vi "Write Return File Path Msg.vi"(10 "Return File Path Msg":refnum<class "Return File Path Msg.lvclass">, 11 "File Dialog in":refnum<class "File Dialog.lvclass">) -> (3 "File Dialog out":refnum<class "File Dialog.lvclass">)   [LabVIEW 2018, in "File Dialog Actor.lvlib" / "File Dialog.lvclass"]
uses:
  File Dialog.lvclass
  File Dialog Messages/Return File Path Msg/Return File Path Msg.lvclass
  File Dialog.lvclass/File Dialog.ctl
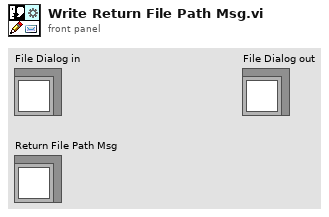
[diagram p1: front panel]
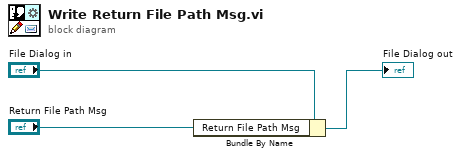
[diagram p0: block diagram]
diagram:
  n1 = Bundle By Name(cluster="File Dialog in", "Return File Path Msg"="Return File Path Msg") -> (→"File Dialog out":refnum<class "File Dialog.lvclass">)
